vi "Create IO Test Configuration.vi"(8 "Error In":errorcluster, 9 "channel classification":T1, 10 "Client Connection Configuration":T2) -> (0 "Error Out":errorcluster, 3 "module":refnum<class "OPC UA Client configuration.lvclass">)   [LabVIEW 2013, in "OPC UA Client Tests.lvlib"]
doc: "Create Client Input test configuration."
uses:
  OPC UA Client Tests.lvlib
  module/configuration/OPC UA Client configuration.lvclass
  module/configuration/Client Connection Configuration.ctl
  <vilib>/NI/Tag Bus Module Framework/channel/channel classification.ctl
  module/configuration/OPC UA Data Type.ctl
  module/configuration/Line.ctl
  <vilib>/NI/Tag Bus Module Framework/channel/TBM channel.lvclass
  module/configuration/OPC UA Client configuration.lvclass/OPC UA Client configuration.ctl
  module/configuration/Write Connection Configuration.vi
  <vilib>/NI/Configuration Framework/serializable configuration/NISE_CEF_serializable configuration.lvclass
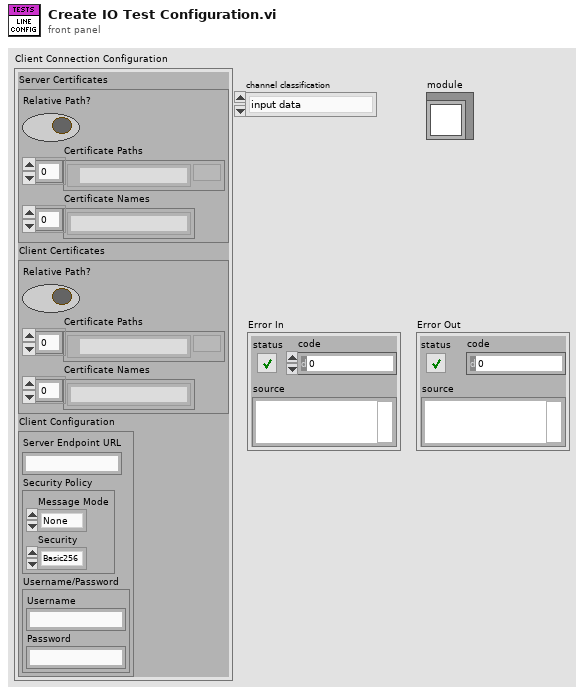
[diagram p1: front panel]
types:
  T1 = typedef "TBM channel.lvclass/channel classification.ctl" = enum16{"input data", "output data", "processing parameter", "processing result"}
  T2 = typedef "OPC UA Client configuration.lvclass/Client Connection Configuration.ctl" = cluster{"Server Certificates":cluster{"Relative Path?":bool, "Certificate Paths":path[], "Certificate Names":string[]}, "Client Certificates":cluster{"Relative Path?":bool, "Certificate Paths":path[], "Certificate Names":string[]}, "Client Configuration":cluster{"Server Endpoint URL":string, "Security Policy":cluster{"Message Mode":enum16{"None", "Sign", "Sign and Encrypt"}, "Security":enum16{"Basic256", "Basic128Rsa15"}}, "Username/Password":cluster{"Username":string, "Password":string}}}
  T3 = typedef "OPC UA Client configuration.lvclass/OPC UA Data Type.ctl" = u16
  T4 = typedef "OPC UA Client configuration.lvclass/Line.ctl" = cluster{"channel":refnum<class "TBM channel.lvclass">, "Node Path":string, "OPC UA Data Type":T3}
  T5 = typedef "tag bus.lvlib/tag descriptor.lvclass/Data Type.ctl" = enum16{"Double", "Single", "I64", "I32", "I16", "I8", "U64", "U32", "U16", "U8", "Boolean", "String", "Array of Double", "Array of Single", "Array of I64", "Array of I32", "Array of I16", "Array of I8", "Array of U64", "Array of U32", "Array of U16", "Array of U8", "Array of Boolean", "Array of String"}
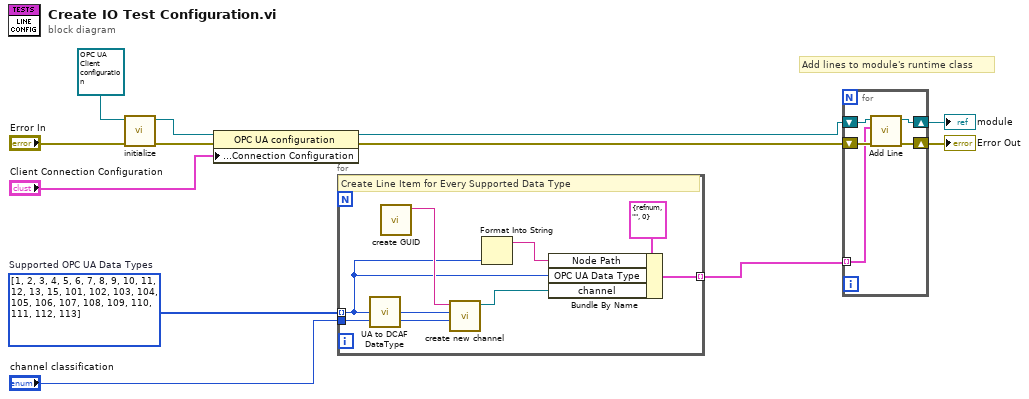
[diagram p0: block diagram]
diagram:
  w3 = T3[] [1, 2, 3, 4, 5, 6, 7, 8, 9, 10, 11, 12, 13, 15, 101, 102, 103, 104, 105, 106, 107, 108, 109, 110, 111, 112, 113] items=["Boolean"=1, "SByte"=2, "Byte"=3, "Int16"=4, "UInt16"=5, "Int32"=6, "UInt32"=7, "Int64"=8, "UInt64"=9, "Float"=10, "Double"=11, "String"=12, "DateTime"=13, "ByteString"=15, "Array of Boolean"=101, "Array of SByte"=102, "Array of Byte"=103, "Array of Int16"=104, "Array of UInt16"=105, "Array of Int32"=106, "Array of UInt32"=107, "Array of Int64"=108, "Array of UInt64"=109, "Array of Float"=110, "Array of Double"=111, "Array of String"=112, "Array of DateTime"=113, "Array of ByteString"=115]  # Supported OPC UA Data Types
  # "Add lines to module's runtime class"
  n1 = call <vilib>:"initialize.vi"("error in"="Error In", "configuration in"=refnum<class "OPC UA Client configuration.lvclass"> refnum ("tag bus configurable plugin module configuration")) -> ("error out"=w11:errorcluster, "configuration out"=w9:refnum<class "OPC UA Client configuration.lvclass">)  [unwired: 7 in, 1 out]
  n2 = property class="OPC UA configuration"(reference=w9, error in=w11, "Customize:Properties:Connection Configuration"="Client Connection Configuration") -> (reference out=w5:refnum<class "OPC UA Client configuration.lvclass">, error out=w10:errorcluster)
  n3 = for {
    tunnel: "channel classification" -> [w20]
    tunnel: [w17] -> w8 mode=indexing
    tunnel: w3 -> [w13] mode=indexing
    # "Create Line Item for Every Supported Data Type"
    n4 = call "UA to DCAF DataType.vi"("OPC UA Data Type"=w13) -> ("DCAF Datatype"=w15:T5)
    n5 = call <vilib>:"create GUID.vi"() -> ("uuid"=w19:string)  [unwired: 10 in, 1 out]
    n6 = call <vilib>:"create new channel.vi"("channel classification"=w20, "data type"=w15, "channel name"=w19) -> ("channel"=w16:refnum<class "TBM channel.lvclass">)  [unwired: 8 in]
    n7 = Format Into String(w13) -> (resulting string=w14:string)  [unwired: 3 in, 1 out]
    n8 = Bundle By Name(cluster=T4 {"channel"=refnum, "Node Path"="", "OPC UA Data Type"=0} ("Line"), "Node Path"=w14, "OPC UA Data Type"=w13, "channel"=w16) -> (w17:T4)
  }
  n9 = for {
    tunnel: w8 -> [w21] mode=indexing
    shift-right: [w24] -> w7
    shift-left: w5 -> [w25]
    shift-right: [w22] -> w12
    shift-left: w10 -> [w23]
    n10 = call "Add Line.vi"("error in"=w23, "Line"=w21, "OPC UA configuration in"=w25) -> ("error out"=w22:errorcluster, "OPC UA configuration out"=w24:refnum<class "OPC UA Client configuration.lvclass">)  [unwired: 7 in]
  }
  "Error Out" <- w12
  "module" <- w7
